vi "Temp Control GUI.vi"(9 "Standalone":bool=TRUE, 10 "Init Data":variant, 11 "Device Name":string="temp control 1") -> ()   [LabVIEW 2024]
uses:
  typedefs/CC enum Operation Mode.ctl
  Subsystems/SS typedef cluster Instrument Command Queue Data.ctl
  Subsystems/SS cluster Data Queue type.ctl
  hk-channel-class/hk-channel-class/HK Item/HK Item.lvclass
  typedefs/CC cluster Alarm Data.ctl
  Temp Control/Temp Control.lvclass
  Current Status/Data Buffer/Data Buffer.lvclass
  typedefs/CC enum Status FG Action.ctl
  Temp Control/Lakeshore 325/Lakeshore 325.lvclass
  Temp Control/Lakeshore 331/Lakeshore 331.lvclass
  Temp Control/Lakeshore 336/Lakeshore 336.lvclass
  Temp Control/Lakeshore 218/Lakeshore 218.lvclass
  typedefs/CC enum Subsystem Status.ctl
  hk-channel-class/hk-channel-class/HK Item/HK Item.lvclass/HK Item.ctl
  hk-channel-class/hk-channel-class/HK Item/HK Channel cluster Telemetry Data.ctl
  hk-channel-class/hk-channel-class/HK Item/HK Channel enum Data Type.ctl
  <vilib>/Utility/error.llb/DialogType.ctl
  hk-channel-class/hk-channel-class/HK Item/Write Source.vi
  6db094d1-7fd6-4988-9962-decbce56bcaa.vi
  40afddd7-fa93-47ab-b467-3e4868690066.vi
panel:
  in  "My Name":string
  in  "Mode":T1
  in  "Tab Control":T2(tab)
  in  "Control enable 2":bool
  in  "Setpoint 2":dbl
  in  "Control enable 1":bool
  in  "Setpoint 1":dbl
  out "Alarm Message":string
  out "Connected":bool
  in  "Status":i32[](listbox)
  out "XY Graph":T3(graph)
  in  "Select Channel":i32=1 min=1 max=4 step=1
  in  "Control Parms":cluster{"P":dbl, "I":dbl, "D":u16}[](array[cluster])
  in  "Reinit":bool
  in  "Heater Range (0: Off)":u16(ring) items=["Off", "Low (0.5W)", "Med (5W)", "High (50W)"]
  in  "Channel Name Prefix":string
  in  "Settings Button":bool
  in  "Power (%)":dbl
  in  "Control Method":bool
  in  "Init Message":string="Connecting to Hardware..."
  in  "Addr":refnum<visa-resource-name>
  in  "Tempcontrol Type":u16(ring) items=["Simulation", "Lakeshore 325", "Lakeshore 336"]
  in  "Close":bool
  out "x-y":u32
  out "Log":string
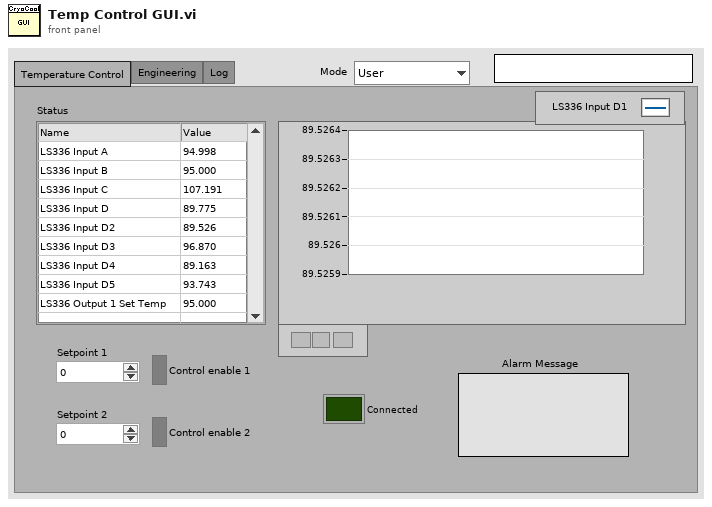
[diagram p1: front panel]
types:
  T1 = typedef "CC enum Operation Mode.ctl" = enum16{"User", "Engineering"}
  T2 = enum32{"Temperature Control", "Engineering", "Log"}
  T3 = cluster{cluster{"Time Stamp":timestamp, "Numeric":dbl}[]}[]
  T4 = typedef "SS typedef cluster Instrument Command Queue Data.ctl" = cluster{"Cmd":string, "Parameters":variant}
  T5 = typedef "CC cluster Alarm Data.ctl" = cluster{"Measured Value":dbl, "Alarm Low":dbl, "Alarm High":dbl, "Message":string, "Source":string}
  T6 = cluster{"state":refnum<user-event>, "cmd q":refnum<queue>, "Cmd":T4, "Data Q":refnum<queue>, "error":errorcluster, "next poll":timestamp, "poll":bool, "Channel List":refnum<class "HK Item.lvclass">[], "Focus Pos":dbl, "Data":dbl[], "Alarm":bool, "Alarms":T5[], "Shutdown":bool, "Device":string, "Temp Control ref":refnum<class "Temp Control.lvclass">, "Buffer":refnum<class "Data Buffer.lvclass">}
  T7 = typedef "CC enum Status FG Action.ctl" = enum16{"Read", "Write", "Init"}
  T8 = typedef "CC enum Subsystem Status.ctl" = enum16{"Unknown", "Ready", "Error"}
  T9 = typedef "SS cluster Data Queue type.ctl" = cluster{"Source":string, "Type":string, "Data":variant}
  T10 = typedef "HK Item.lvclass/HK Channel enum Data Type.ctl" = enum16{"Floating Point", "Integer", "Enum", "String", "Waveform", "File"}
  T11 = typedef "HK Item.lvclass/HK Channel cluster Telemetry Data.ctl" = cluster{"Ch Names":string[], "Ch Values":dbl[], "Timestamp":timestamp, "Data Type":T10}
  T12 = typedef "CC cluster Device Index.ctl" = cluster{"Device Type Name":string, "Curr Device Name":string, "All Instances":string[]}
  T13 = typedef "HK Item.lvclass/HK Channel Units and Setup.ctl" = cluster{"Unit Type":string, "Units":string, "Configuration":string, "Digits":i32, "Data Type":T10, "Exponential?":bool, "Source":string}
  T14 = cluster{cluster{"Time Stamp":timestamp, "Numeric":dbl}[]}
  T15 = typedef "DialogType.ctl" = u16
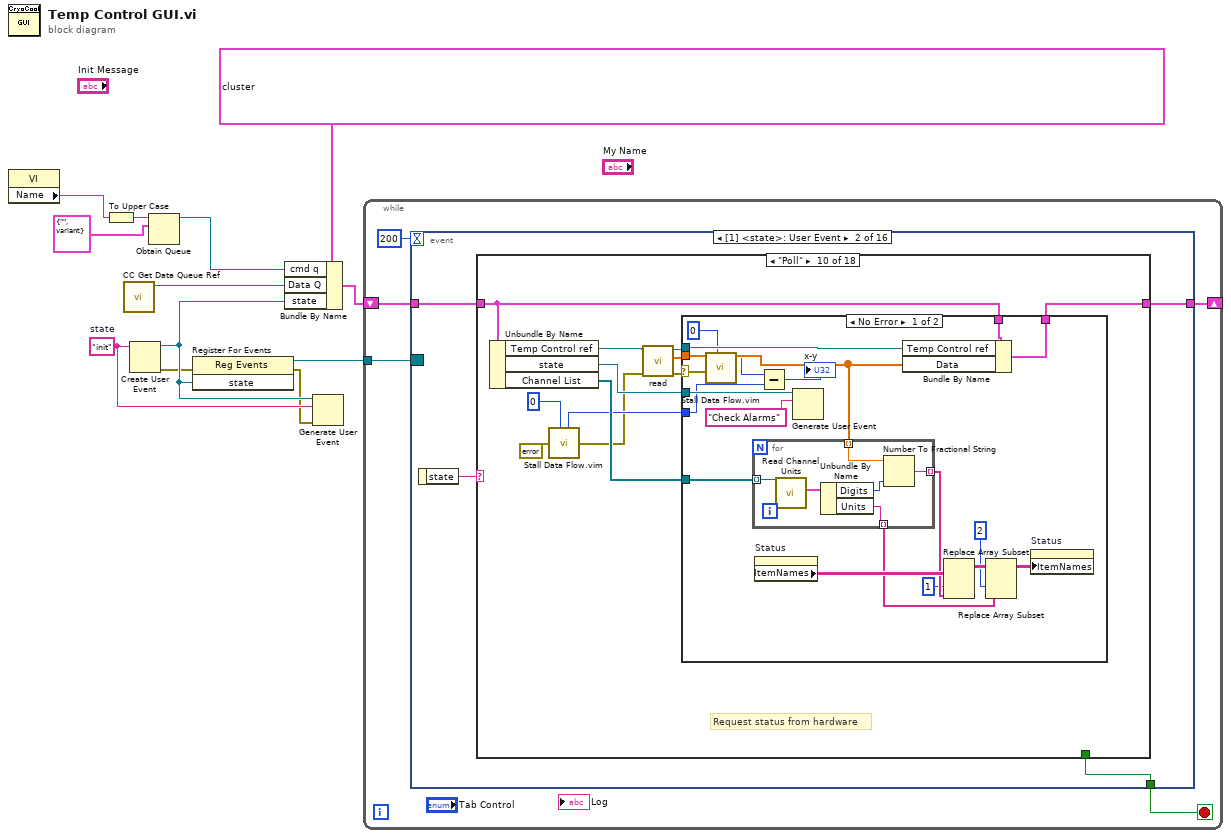
[diagram p0: block diagram]
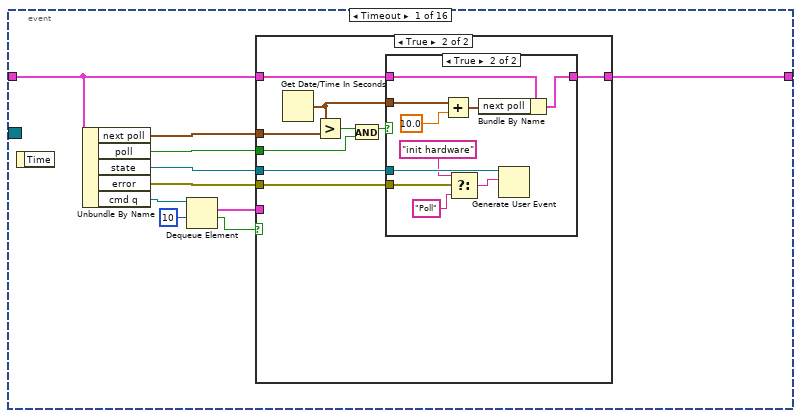
[diagram p2: hidden frame]
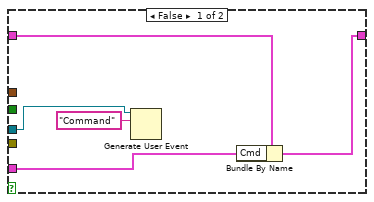
[diagram p3: hidden frame]
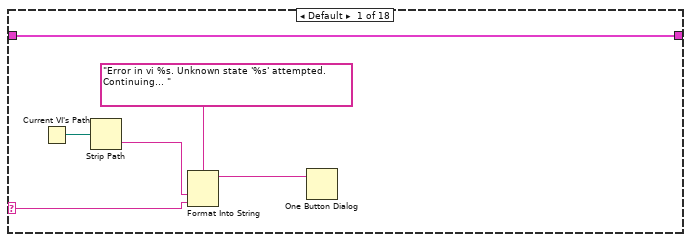
[diagram p5: hidden frame]
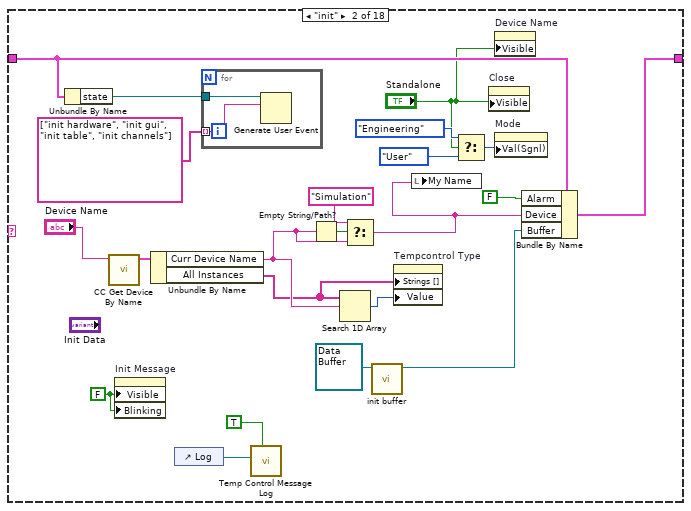
[diagram p6: hidden frame]
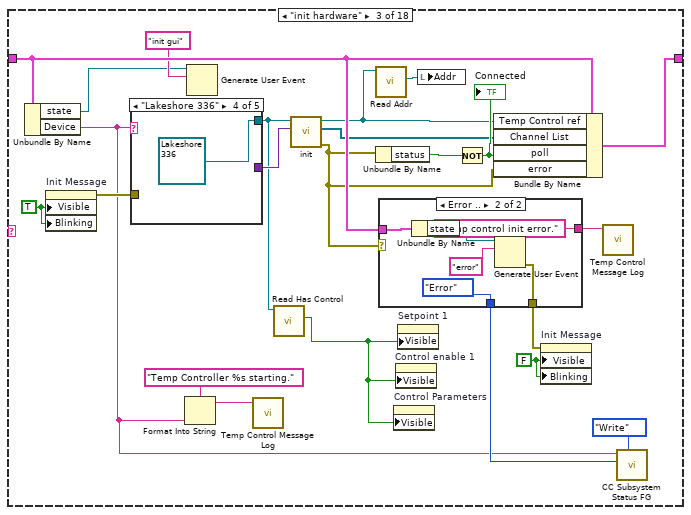
[diagram p7: hidden frame]
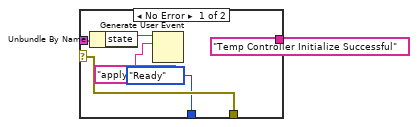
[diagram p8: hidden frame]
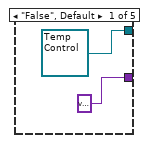
[diagram p9: hidden frame]
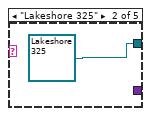
[diagram p10: hidden frame]
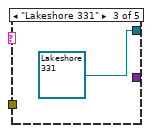
[diagram p11: hidden frame]
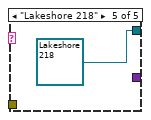
[diagram p12: hidden frame]
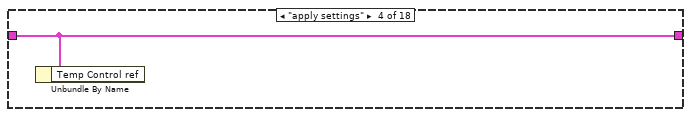
[diagram p13: hidden frame]
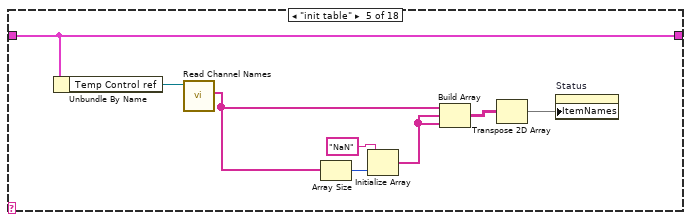
[diagram p14: hidden frame]
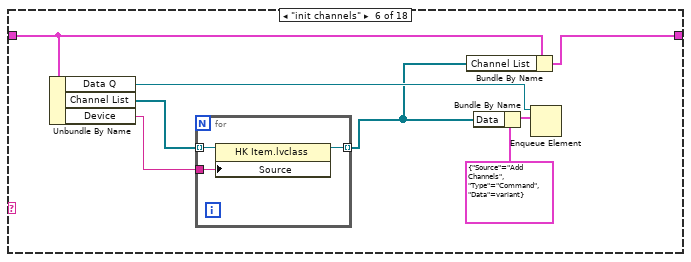
[diagram p15: hidden frame]
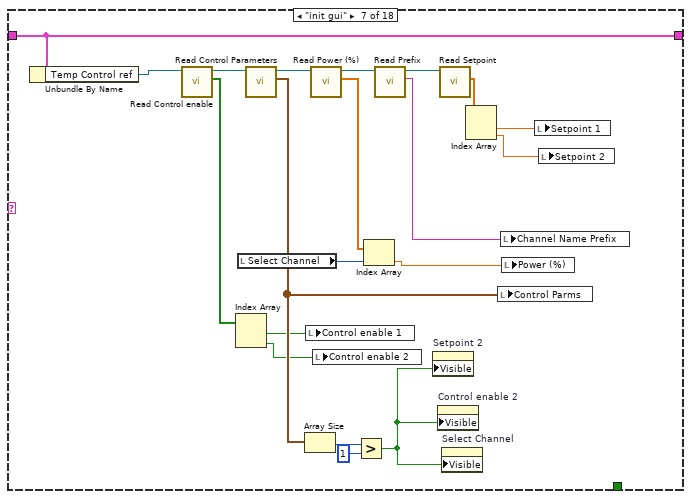
[diagram p16: hidden frame]
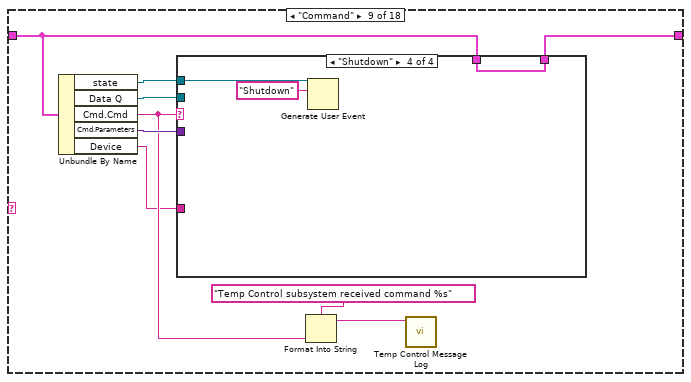
[diagram p18: hidden frame]
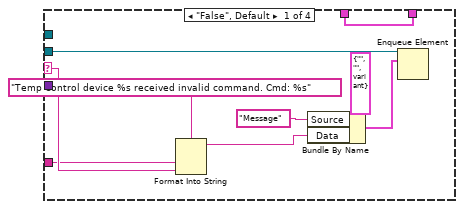
[diagram p19: hidden frame]
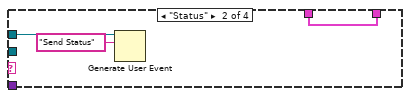
[diagram p20: hidden frame]
diagram:
  w8 = "init"  # state
  n1 = property class="VI"() -> ("Name"=w1:string)  [unwired: 2 in, 2 out]
  n2 = To Upper Case(1:w1) -> (0:w4:string)
  n3 = call "CC Get Data Queue Ref.vi"() -> ("Data Q"=w5:refnum<queue>)  [unwired: 10 in, 1 out]
  n4 = Create User Event(user event datatype=w8) -> (user event=w10:refnum<user-event>, error out=w6:errorcluster)  [unwired: 1 in]
  n5 = Obtain Queue(name (unnamed)=w4, element data type=T4 {"Cmd"="", "Parameters"=variant}) -> (queue out=w2:refnum<queue>)  [unwired: 3 in, 2 out]
  n6 = register-events(error in=w6, w10) -> (reference out=w9:refnum<event-registration>, error out=w7:errorcluster)  [unwired: 1 in]
  n7 = Bundle By Name(cluster=T6 {"state"=refnum, "cmd q"=refnum, "Cmd"={"Cmd"="", "Parameters"=variant}, "Data Q"=refnum, "error"={"status"=FALSE, "code"=0, "source"=""}, "next poll"=timestamp(0 s since 1904-01-01), "poll"=FALSE, "Channel List"=[], "Focus Pos"=0.0, "Data"=[], "Alarm"=FALSE, "Alarms"=[], "Shutdown"=FALSE, "Device"="", "Temp Control ref"=refnum, "Buffer"=refnum}, "cmd q"=w2, "Data Q"=w5, "state"=w10) -> (w11:T6)
  n8 = Generate User Event(user event=w10, event data cluster=w8, error in=w7) -> ()  [unwired: 1 in, 2 out]
  n9 = while {
    tunnel: w9 -> [w17]
    shift-right: [w15] -> _
    shift-left: w11 -> [w16]
    stop <- w14 stop-if-true
    n10 = event shown="[1] <state>: User Event" {
      selector: w17 -> [_ _ _ _ _ _ _ _ _ _ _ _ _ _ _ _]
      dyn-events: _ -> [_ _ _ _ _ _ _ _ _ _ _ _ _ _ _ _]
      timeout: 200 -> [_ _ _ _ _ _ _ _ _ _ _ _ _ _ _ _]
      tunnel: w16 -> [w22 w55 w314 w318 w323 w333 w345 w358 w374 w381 w382 w406 w411 w418 w424 w431]
      tunnel: [w21 w54 w314 w319 w324 w334 w346 w359 w375 w381 w383 w407 w412 w418 w424 w431] -> w15
      tunnel: [_ w53 _ _ _ _ _ _ _ _ _ _ _ _ _ _] -> w14
      event Timeout {
        n11 = event-data() -> ()  [unwired: 1 in, 1 out]
        n12 = Unbundle By Name(w22) -> ("next poll"=w20:timestamp, "poll"=w19:bool, "state"=w23:refnum<user-event>, "error"=w18:errorcluster, "cmd q"=w27:refnum<queue>)
        n13 = Dequeue Element(queue=w27, timeout in ms (-1)=10) -> (element=w24:T4, timed out?=w25:bool)  [unwired: 1 in, 2 out]
        n14 = case shown="True" w25 {
          tunnel: w24 -> [w29 _]
          tunnel: w23 -> [w32 w38]
          tunnel: w22 -> [w30 w39]
          tunnel: [w28 w36] -> w21
          tunnel: w20 -> [_ w41]
          tunnel: w19 -> [_ w34]
          tunnel: w18 -> [_ w33]
          frame False {
            n15 = Generate User Event(user event=w32, event data cluster="Command" ("event data")) -> ()  [unwired: 2 in, 2 out]
            n16 = Bundle By Name(cluster=w30, "Cmd"=w29) -> (w28:T6)
          }
          frame True {
            n17 = Get Date/Time In Seconds() -> (seconds since 1Jan1904=w37:timestamp)
            n18 = Greater?(x=w37, y=w41) -> (0:w40:bool)
            n19 = And(x=w40, y=w34) -> (x .and. y?=w35:bool)
            n20 = case shown="True" w35 {
              tunnel: w39 -> [w42 w52]
              tunnel: w38 -> [_ w51]
              tunnel: w37 -> [_ w50]
              tunnel: [w42 w47] -> w36
              tunnel: w33 -> [_ w45]
              frame False {
              }
              frame True {
                n21 = Add(x=w50, y=10.0) -> (x+y=w48:timestamp)
                n22 = Select(t="init hardware", s=w45, f="Poll" ("event data")) -> (s? t:f=w43:string)
                n23 = Bundle By Name(cluster=w52, "next poll"=w48) -> (w47:T6)
                n24 = Generate User Event(user event=w51, event data cluster=w43) -> ()  [unwired: 2 in, 2 out]
              }
            }
          }
        }
      }
      event User Event {
        n25 = event-data() -> ("state"=w56:string)  [unwired: 1 in]
        n26 = case shown="\"Poll\"" w56 {
          selector: w56 -> [w61 _ _ _ _ _ _ _ _ _ _ _ _ _ _ _ _ _]
          tunnel: w55 -> [w57 w82 w106 w128 w136 w138 w167 w168 w173 w206 w239 w245 w253 w258 w275 w282 w286 w310]
          tunnel: [w57 w83 w109 w128 w136 w139 w167 w168 w174 w207 w239 w245 w253 w258 w275 w283 w287 w310] -> w54
          tunnel: [_ _ _ _ _ _ _ _ _ _ _ _ _ _ _ _ _ TRUE] -> w53
          frame Default {
            n27 = Current VI's Path() -> (path=w60:path)
            n28 = Strip Path(path=w60) -> (name=w59:string)  [unwired: 1 out]
            n29 = Format Into String(format string="Error in vi %s. Unknown state '%s' attempted. Continuing... ", w59, w61) -> (resulting string=w58:string)  [unwired: 2 in, 1 out]
            n30 = One Button Dialog(message=w58) -> ()  [unwired: 1 in, 1 out]
          }
          frame "init" {
            w69 = FALSE ("Visible")
            n31 = Unbundle By Name(w82) -> ("state"=w81:refnum<user-event>)
            n32 = call "CC Get Device By Name.vi"("Device Type"="Device Name") -> ("Device"=w77:T12)  [unwired: 8 in, 2 out]
            n33 = property on="Init Message" class="Str"("Visible"=w69, "Blinking"=w69) -> ()  [unwired: 2 in, 2 out]
            n34 = Unbundle By Name(w77) -> ("Curr Device Name"=w76:string, "All Instances"=w75:string[])
            n35 = control-ref of="Log"() -> (w71:refnum<vi>)
            n36 = for {
              tunnel: w81 -> [w86]
              tunnel: string[] ["init hardware", "init gui", "init table", "init channels"] -> [w85] mode=indexing
              n37 = Generate User Event(user event=w86, event data cluster=w85) -> ()  [unwired: 2 in, 2 out]
            }
            n38 = call "Temp Control Message Log.vi"("init?"=TRUE, "Log Ref"=w71) -> ()  [unwired: 8 in, 2 out]
            n39 = Empty String/Path?(string/path=w76) -> (empty?=w84:bool)
            n40 = Search 1D Array(1D array=w75, element=w76) -> (index of element=w79:i32)  [unwired: 1 in]
            n41 = Select(t="Simulation", s=w84, f=w76) -> (s? t:f=w67:string)
            n42 = call-dynamic "init buffer.vi"("Data Buffer in"=refnum<class "Data Buffer.lvclass"> refnum) -> ("Data Buffer out"=w65:refnum<class "Data Buffer.lvclass">)  [unwired: 9 in, 1 out]
            n43 = property on="Tempcontrol Type" class="Ring (strict)"("Strings []"=w75, "Value"=w79) -> ()  [unwired: 2 in, 2 out]
            n44 = local write "My Name"(w67) -> ()
            n45 = Select(t=CC_enum_Operation_Mode."Engineering" ("Mode"), s="Standalone", f=CC_enum_Operation_Mode."User" ("Mode")) -> (s? t:f=w72:T1)
            n46 = property on="Close" class="Bool"("Visible"="Standalone") -> ()  [unwired: 2 in, 2 out]
            n47 = property on="Device Name" class="Str"("Visible"="Standalone") -> ()  [unwired: 2 in, 2 out]
            n48 = property on="Mode" class="Enum (strict)"("Val(Sgnl)"=w72) -> ()  [unwired: 2 in, 2 out]
            n49 = Bundle By Name(cluster=w82, "Alarm"=FALSE, "Device"=w67, "Buffer"=w65) -> (w83:T6)
          }
          frame "init hardware" {
            w101 = FALSE ("Visible")
            w103 = TRUE ("Visible")
            n50 = Unbundle By Name(w106) -> ("state"=w87:refnum<user-event>, "Device"=w94:string)
            n51 = property on="Init Message" class="Str"("Visible"=w103, "Blinking"=w103) -> (error out=w102:errorcluster)  [unwired: 2 in, 1 out]
            n52 = case shown="\"Lakeshore 336\"" w94 {
              tunnel: [refnum<class "Temp Control.lvclass"> refnum ("Temp Control.lvclass") refnum<class "Lakeshore 325.lvclass"> refnum ("Lakeshore 325.lvclass") refnum<class "Lakeshore 331.lvclass"> refnum ("Lakeshore 331.lvclass") refnum<class "Lakeshore 336.lvclass"> refnum ("Lakeshore 336.lvclass") refnum<class "Lakeshore 218.lvclass"> refnum ("Lakeshore 218.lvclass")] -> w91
              tunnel: [variant _ _ _ _] -> w95
              tunnel: w102 -> [_ _ _ _ _]
              frame "False", Default {
              }
              frame "Lakeshore 325" {
              }
              frame "Lakeshore 331" {
              }
              frame "Lakeshore 336" {
              }
              frame "Lakeshore 218" {
              }
            }
            n53 = Format Into String(format string="Temp Controller %s starting.", w94) -> (resulting string=w104:string)  [unwired: 2 in, 1 out]
            n54 = Generate User Event(user event=w87, event data cluster="init gui" ("event data")) -> ()  [unwired: 2 in, 2 out]
            n55 = call "Temp Control Message Log.vi"("String in"=w104) -> ()  [unwired: 9 in, 2 out]
            n56 = call-dynamic "Read Has Control.vi"("Temp Control in"=w91) -> ("Has Control"=w90:bool)  [unwired: 8 in, 2 out]
            n57 = call-dynamic "init.vi"("Init Data"=w95, "Temp Control in"=w91) -> ("error out"=w96:errorcluster, "Channel List"=w97:refnum<class "HK Item.lvclass">[], "Temp Control out"=w92:refnum<class "Temp Control.lvclass">)  [unwired: 7 in]
            n58 = call-dynamic "Read Addr.vi"("Temp Control in"=w92) -> ("Addr"=w93:refnum<visa-resource-name>)  [unwired: 8 in, 2 out]
            n59 = Unbundle By Name(w96) -> ("status"=w108:bool)
            n60 = case shown="Error .." w96 {
              selector: w96 -> [w115 _]
              tunnel: w106 -> [w112 w121]
              tunnel: [w115 w118] -> w100
              tunnel: [CC_enum_Subsystem_Status."Ready" ("Status") CC_enum_Subsystem_Status."Error" ("Status")] -> w98
              tunnel: ["Temp Controller Initialize Successful" ("String in") "Temp control init error." ("String in")] -> w88
              frame No Error {
                n61 = Unbundle By Name(w112) -> ("state"=w111:refnum<user-event>)
                n62 = Generate User Event(user event=w111, event data cluster="apply settings" ("event data")) -> ()  [unwired: 2 in, 2 out]
              }
              frame Error {
                n63 = Unbundle By Name(w121) -> ("state"=w120:refnum<user-event>)
                n64 = Generate User Event(user event=w120, event data cluster="error" ("event data")) -> (error out=w118:errorcluster)  [unwired: 2 in, 1 out]
              }
            }
            n65 = property on="Control Parameters" class="Clust (strict)"("Visible"=w90) -> ()  [unwired: 2 in, 2 out]
            n66 = property on="Control enable 1" class="Bool (strict)"("Visible"=w90) -> ()  [unwired: 2 in, 2 out]
            n67 = property on="Setpoint 1" class="DigNum (strict)"("Visible"=w90) -> ()  [unwired: 2 in, 2 out]
            n68 = local write "Addr"(w93) -> ()
            n69 = Not(x=w108) -> (.not. x?=w105:bool)
            "Connected" <- w105
            n70 = Bundle By Name(cluster=w106, "Temp Control ref"=w92, "Channel List"=w97, "poll"=w105, "error"=w96) -> (w109:T6)
            n71 = property on="Init Message" class="Str"(error in=w100, "Visible"=w101, "Blinking"=w101) -> ()  [unwired: 1 in, 2 out]
            n72 = call "Temp Control Message Log.vi"("String in"=w88) -> ()  [unwired: 9 in, 2 out]
            n73 = call "CC Subsystem Status FG.vi"("Action"=CC_enum_Status_FG_Action."Write", "Status"=w98, "Subsystem Name"=w94) -> ()  [unwired: 7 in, 2 out]
          }
          frame "apply settings" {
            n74 = Unbundle By Name(w128) -> ()  [unwired: 1 out]
          }
          frame "init table" {
            n75 = Unbundle By Name(w136) -> ("Temp Control ref"=w130:refnum<class "Temp Control.lvclass">)
            n76 = call-dynamic "Read Channel Names.vi"("Temp Control in"=w130) -> ("Channel Names"=w129:string[])  [unwired: 8 in, 2 out]
            n77 = Array Size(array=w129) -> (size(s)=w135:i32)
            n78 = Initialize Array("NaN", w135) -> (w131:string[])
            n79 = Build Array(w129, w131, w131) -> (w133:string[][])
            n80 = Transpose 2D Array(2D array=w133) -> (transposed array=w132:string[][])
            n81 = property on="Status" class="MCListbox (strict)"("ItemNames"=w132) -> ()  [unwired: 2 in, 2 out]
          }
          frame "init channels" {
            n82 = Unbundle By Name(w138) -> ("Data Q"=w142:refnum<queue>, "Channel List"=w141:refnum<class "HK Item.lvclass">[], "Device"=w137:string)
            n83 = for {
              tunnel: w141 -> [w147] mode=indexing
              tunnel: [w146] -> w140 mode=indexing
              tunnel: w137 -> [w145]
              n84 = property class="HK Item.lvclass"(reference=w147, "Source"=w145) -> (reference out=w146:refnum<class "HK Item.lvclass">)  [unwired: 1 in, 1 out]
            }
            n85 = Bundle By Name(cluster=w138, "Channel List"=w140) -> (w139:T6)
            n86 = Bundle By Name(cluster=T9 {"Source"="Add Channels", "Type"="Command", "Data"=variant} ("element"), "Data"=w140) -> (w144:T9)
            n87 = Enqueue Element(queue=w142, element=w144) -> ()  [unwired: 2 in, 3 out]
          }
          frame "init gui" {
            n88 = Unbundle By Name(w167) -> ("Temp Control ref"=w166:refnum<class "Temp Control.lvclass">)
            n89 = call-dynamic "Read Control enable.vi"("Temp Control in"=w166) -> ("Control Enable"=w160:bool[], "Temp Control out"=w165:refnum<class "Temp Control.lvclass">)  [unwired: 8 in, 1 out]
            n90 = Index Array(array=w160) -> (element #1=w154:bool, element #2=w148:bool)  [unwired: 2 in]
            n91 = local read "Select Channel"() -> (w150:i32)
            n92 = call-dynamic "Read Control Parameters.vi"("Temp Control in"=w165) -> ("Control Parameters"=w158:cluster{"P":dbl, "I":dbl, "D":u16}[], "Temp Control out"=w164:refnum<class "Temp Control.lvclass">)  [unwired: 8 in, 1 out]
            n93 = Array Size(array=w158) -> (size(s)=w157:i32)
            n94 = local write "Control enable 1"(w154) -> ()
            n95 = call-dynamic "Read Power (%).vi"("Temp Control in"=w164) -> ("Power (%)"=w153:dbl[], "Temp Control out"=w163:refnum<class "Temp Control.lvclass">)  [unwired: 8 in, 1 out]
            n96 = local write "Control enable 2"(w148) -> ()
            n97 = Greater?(x=w157, y=1) -> (0:w155:bool)
            n98 = Index Array(array=w153, index=w150) -> (element=w152:dbl)
            n99 = call-dynamic "Read Prefix.vi"("Temp Control in"=w163) -> ("Prefix"=w161:string, "Temp Control out"=w162:refnum<class "Temp Control.lvclass">)  [unwired: 8 in, 1 out]
            n100 = property on="Setpoint 2" class="DigNum (strict)"("Visible"=w155) -> ()  [unwired: 2 in, 2 out]
            n101 = property on="Control enable 2" class="Bool (strict)"("Visible"=w155) -> ()  [unwired: 2 in, 2 out]
            n102 = call-dynamic "Read Setpoint.vi"("Temp Control in"=w162) -> ("Setpoint"=w159:dbl[])  [unwired: 8 in, 2 out]
            n103 = property on="Select Channel" class="DigNum (strict)"("Visible"=w155) -> ()  [unwired: 2 in, 2 out]
            n104 = Index Array(array=w159) -> (element #1=w151:dbl, element #2=w149:dbl)  [unwired: 2 in]
            n105 = local write "Control Parms"(w158) -> ()
            n106 = local write "Channel Name Prefix"(w161) -> ()
            n107 = local write "Power (%)"(w152) -> ()
            n108 = local write "Setpoint 1"(w151) -> ()
            n109 = local write "Setpoint 2"(w149) -> ()
          }
          frame "send command" {
          }
          frame "Command" {
            n110 = Unbundle By Name(w173) -> ("state"=w175:refnum<user-event>, "Data Q"=w177:refnum<queue>, "Cmd.Cmd"=w171:string, "Cmd.Parameters"=w176:variant, "Device"=w169:string)
            n111 = case shown="\"Shutdown\"" w171 {
              selector: w171 -> [w179 _ _ _]
              tunnel: w177 -> [w186 _ _ _]
              tunnel: w176 -> [_ _ _ _]
              tunnel: w175 -> [_ w189 w191 w195]
              tunnel: w173 -> [w180 w187 w190 w193]
              tunnel: [w180 w187 w190 w193] -> w174
              tunnel: w169 -> [w178 _ _ _]
              frame "False", Default {
                n112 = Format Into String(format string="Temp Control device %s received invalid command. Cmd: %s", w178, w179) -> (resulting string=w182:string)  [unwired: 2 in, 1 out]
                n113 = Bundle By Name(cluster=T9 {"Source"="", "Type"="", "Data"=variant} ("element"), "Source"="Message" ("Data Type"), "Data"=w182) -> (w181:T9)
                n114 = Enqueue Element(queue=w186, element=w181) -> ()  [unwired: 2 in, 3 out]
              }
              frame "Status" {
                n115 = Generate User Event(user event=w189, event data cluster="Send Status" ("event data")) -> ()  [unwired: 2 in, 2 out]
              }
              frame "Config" {
                n116 = Generate User Event(user event=w191, event data cluster="Send Config" ("event data")) -> ()  [unwired: 2 in, 2 out]
              }
              frame "Shutdown" {
                n117 = Generate User Event(user event=w195, event data cluster="Shutdown" ("event data")) -> ()  [unwired: 2 in, 2 out]
              }
            }
            n118 = Format Into String(format string="Temp Control subsystem received command %s", w171) -> (resulting string=w170:string)  [unwired: 2 in, 1 out]
            n119 = call "Temp Control Message Log.vi"("String in"=w170) -> ()  [unwired: 9 in, 2 out]
          }
          frame "Poll" {
            # "Request status from hardware"
            n120 = Unbundle By Name(w206) -> ("Temp Control ref"=w200:refnum<class "Temp Control.lvclass">, "state"=w205:refnum<user-event>, "Channel List"=w204:refnum<class "HK Item.lvclass">[])
            n121 = call "Stall Data Flow.vim"("value in"=errorcluster {"status"=FALSE, "code"=0, "source"=""} ("error in (no error)"), "milliseconds to wait"=u32 0) -> ("millisecond timer value"=w201:u32, "value out"=w199:errorcluster)
            n122 = call-dynamic "read.vi"("error in (no error)"=w199, "Temp Control in"=w200) -> ("error out"=w196:errorcluster, "Data"=w197:dbl[], "Temp Control out"=w198:refnum<class "Temp Control.lvclass">)  [unwired: 7 in]
            n123 = case shown="No Error" w196 {
              selector: w196 -> [w216 w234]
              tunnel: [w226 w233] -> w207
              tunnel: w206 -> [w225 w235]
              tunnel: w205 -> [w224 w237]
              tunnel: w198 -> [w222 _]
              tunnel: w204 -> [w221 _]
              tunnel: w197 -> [w220 _]
              tunnel: w201 -> [w213 _]
              frame No Error {
                n124 = call "Stall Data Flow.vim"("value in"=w216, "milliseconds to wait"=u32 0) -> ("millisecond timer value"=w214:u32)  [unwired: 1 out]
                n125 = for {
                  tunnel: w221 -> [w232] mode=indexing
                  tunnel: w220 -> [w229] mode=indexing
                  tunnel: [w228] -> w218 mode=indexing
                  tunnel: [w227] -> w209 mode=indexing
                  n126 = call "Read Channel Units.vi"("HK Item in"=w232) -> ("Channel Setup"=w231:T13)  [unwired: 8 in, 2 out]
                  n127 = Unbundle By Name(w231) -> ("Digits"=w230:i32, "Units"=w227:string)
                  n128 = Number To Fractional String(number=w229, precision (6)=w230) -> (F-format string=w228:string)  [unwired: 2 in]
                }
                n129 = property on="Status" class="MCListbox (strict)"() -> ("ItemNames"=w219:string[][])  [unwired: 2 in, 2 out]
                n130 = Subtract(x=w214, y=w213) -> (x-y=→"x-y":u32)
                n131 = Generate User Event(user event=w224, event data cluster="Check Alarms" ("event data")) -> ()  [unwired: 2 in, 2 out]
                n132 = Bundle By Name(cluster=w225, "Temp Control ref"=w222, "Data"=w220) -> (w226:T6)
                n133 = Replace Array Subset(array=w219, new element=w218, index (col)=1 ("disabled index (col)")) -> (w211:string[][])  [unwired: 1 in]
                n134 = Replace Array Subset(array=w211, new element=w209, index (col)=2 ("disabled index (col)")) -> (w208:string[][])  [unwired: 1 in]
                n135 = property on="Status" class="MCListbox (strict)"("ItemNames"=w208) -> ()  [unwired: 2 in, 2 out]
              }
              frame Error {
                n136 = Generate User Event(user event=w237, event data cluster="error" ("event data")) -> ()  [unwired: 2 in, 2 out]
                n137 = Bundle By Name(cluster=w235, "error"=w234) -> (w233:T6)
              }
            }
          }
          frame "Check Alarms" {
            n138 = Unbundle By Name(w239) -> ("state"=w238:refnum<user-event>)
            n139 = Generate User Event(user event=w238, event data cluster="Send Status" ("event data")) -> ()  [unwired: 2 in, 2 out]
          }
          frame "Alarm Set" {
            n140 = Unbundle By Name(w245) -> ("Data Q"=w250:refnum<queue>, "Device"=w242:string, "Alarms"=w247:T5[])
            n141 = Index Array(array=w247) -> (element=w246:T5)  [unwired: 1 in]
            n142 = Bundle By Name(cluster=w246, "Source"=w242) -> (w243:T5)
            n143 = Unbundle By Name(w243) -> ("Message"=w244:string)
            "Alarm Message" <- w244
            n144 = Bundle By Name(cluster=T9 {"Source"="", "Type"="", "Data"=variant} ("element"), "Source"=w242, "Type"="Alarm Set", "Data"=w243) -> (w241:T9)
            n145 = Enqueue Element(queue=w250, element=w241) -> ()  [unwired: 2 in, 3 out]
            n146 = call "Temp Control Message Log.vi"("String in"=w244) -> ()  [unwired: 9 in, 2 out]
          }
          frame "Alarm Clear" {
            n147 = Unbundle By Name(w253) -> ("Data Q"=w257:refnum<queue>, "Device"=w254:string)
            n148 = Bundle By Name(cluster=T9 {"Source"="", "Type"="", "Data"=variant} ("element"), "Source"=w254, "Type"="Alarm Clear") -> (w251:T9)
            n149 = call "Temp Control Message Log.vi"("String in"="Alarm condition cleared.") -> ()  [unwired: 9 in, 2 out]
            n150 = Enqueue Element(queue=w257, element=w251) -> ()  [unwired: 2 in, 3 out]
          }
          frame "Alarm Shutdown" {
          }
          frame "Send Status" {
            n151 = Unbundle By Name(w275) -> ("Data Q"=w274:refnum<queue>, "Device"=w264:string, "Temp Control ref"=w263:refnum<class "Temp Control.lvclass">, "Data"=w260:dbl[], "Buffer"=w261:refnum<class "Data Buffer.lvclass">)
            n152 = call-dynamic "Read Channel Names.vi"("Temp Control in"=w263) -> ("Channel Names"=w262:string[])  [unwired: 8 in, 2 out]
            n153 = Get Date/Time In Seconds() -> (seconds since 1Jan1904=w267:timestamp)
            n154 = call-dynamic "write buffer.vi"("Data"=w260, "Data Buffer in"=w261) -> ("XY Graph"=w259:T3)  [unwired: 7 in, 2 out]
            n155 = Bundle(cluster=T11 {"Ch Names"=[], "Ch Values"=[], "Timestamp"=timestamp(0 s since 1904-01-01), "Data Type"=enum."Floating Point"}, "Ch Names"=w262, "Ch Values"=w260, "Timestamp"=w267, "Data Type"=HK_Channel_enum_Data_Type."Floating Point") -> (w269:T11)
            n156 = for {
              tunnel: "Status" -> [w277] mode=indexing
              tunnel: w259 -> [w278]
              tunnel: [w276] -> w265 mode=indexing
              n157 = Index Array(array=w278, index=w277) -> (element=w276:T14)
            }
            "XY Graph" <- w265
            n158 = Bundle By Name(cluster=T9 {"Source"="", "Type"="", "Data"=variant} ("element"), "Source"=w264, "Type"="Floating Point" ("Data Type"), "Data"=w269) -> (w271:T9)
            n159 = Enqueue Element(queue=w274, element=w271) -> ()  [unwired: 2 in, 3 out]
          }
          frame "Reinit" {
            n160 = Unbundle By Name(w282) -> ("Temp Control ref"=w281:refnum<class "Temp Control.lvclass">, "state"=w285:refnum<user-event>)
            n161 = call-dynamic "close.vi"("Temp Control in"=w281) -> ("error out"=w279:errorcluster, "Temp Control out"=w280:refnum<class "Temp Control.lvclass">)  [unwired: 9 in]
            n162 = Generate User Event(user event=w285, event data cluster="init hardware" ("event data")) -> ()  [unwired: 2 in, 2 out]
            n163 = call <vilib>:"Clear Errors.vi"("error in (no error)"=w279) -> ()  [unwired: 5 in, 2 out]
            n164 = Bundle By Name(cluster=w282, "Temp Control ref"=w280) -> (w283:T6)
          }
          frame "error" {
            w299 = T15 0 items=["no dialog", "OK message", "continue or stop message", "OK message + warnings", "continue/stop + warnings"] ("type of dialog (OK msg:1)")
            n165 = Unbundle By Name(w286) -> ("Device"=w291:string, "error"=w302:errorcluster, "error.code"=w305:i32, "error.source"=w303:string, "Data Q"=w293:refnum<queue>)
            n166 = call <vilib>:"Simple Error Handler.vi"("type of dialog (OK msg:1)"=w299, "error in (no error)"=w302) -> ("message"=w301:string)  [unwired: 3 in, 4 out]
            n167 = Bundle By Name(cluster=T5 {"Measured Value"=0.0, "Alarm Low"=0.0, "Alarm High"=0.0, "Message"="", "Source"=""} ("element"), "Source"=w291, "Message"="Temp Controller Initialization Error. Check Communications port.") -> (w295:T5)
            n168 = Format Into String(format string="Error from Temperature Controller \"%s\". Error # %d, Error Source: %s, Error message \"%s\"", w291, w305, w303, w301) -> (resulting string=w300:string)  [unwired: 2 in, 1 out]
            n169 = Bundle By Name(cluster=T9 {"Source"="", "Type"="", "Data"=variant} ("element"), "Source"=w291, "Type"="Alarm Set", "Data"=w295) -> (w292:T9)
            n170 = call "Temp Control Message Log.vi"("String in"=w300) -> ()  [unwired: 9 in, 2 out]
            n171 = Get Date/Time In Seconds() -> (seconds since 1Jan1904=w290:timestamp)
            n172 = Add(x=w290, y=120.0) -> (x+y=w288:timestamp)
            n173 = Enqueue Element(queue=w293, element=w292) -> ()  [unwired: 2 in, 3 out]
            n174 = Bundle By Name(cluster=w286, "next poll"=w288) -> (w287:T6)
          }
          frame "Shutdown" {
            n175 = Unbundle By Name(w310) -> ("Data Q"=w309:refnum<queue>, "Temp Control ref"=w307:refnum<class "Temp Control.lvclass">)
            n176 = Release Queue(queue=w309) -> ()  [unwired: 2 in, 3 out]
            n177 = call-dynamic "close.vi"("Temp Control in"=w307) -> ("error out"=w306:errorcluster)  [unwired: 9 in, 1 out]
            n178 = call <vilib>:"Clear Errors.vi"("error in (no error)"=w306) -> ()  [unwired: 5 in, 2 out]
            n179 = call "Temp Control Message Log.vi"("String in"="Temp Control shutting down.") -> ()  [unwired: 9 in, 2 out]
          }
        }
      }
      event "Select Channel": Value Change {
        n180 = event-data() -> ()  [unwired: 1 in, 1 out]
        n181 = Unbundle By Name(w314) -> ("state"=w313:refnum<user-event>)
        n182 = Generate User Event(user event=w313, event data cluster="init gui" ("event data")) -> ()  [unwired: 2 in, 2 out]
      }
      event "Channel Name Prefix": Value Change {
        n183 = event-data() -> ()  [unwired: 1 in, 6 out]
        n184 = Unbundle By Name(w318) -> ("Temp Control ref"=w321:refnum<class "Temp Control.lvclass">)
        n185 = call-dynamic "Write Prefix.vi"("Prefix"="Channel Name Prefix", "Temp Control in"=w321) -> ("Temp Control out"=w317:refnum<class "Temp Control.lvclass">)  [unwired: 8 in, 1 out]
        n186 = call-dynamic "Read Channel List.vi"("Temp Control in"=w317) -> ("Channel List"=w315:refnum<class "HK Item.lvclass">[], "Temp Control out"=w316:refnum<class "Temp Control.lvclass">)  [unwired: 8 in, 1 out]
        n187 = Bundle By Name(cluster=w318, "Temp Control ref"=w316, "Channel List"=w315) -> (w319:T6)
      }
      event "Control Parms": Value Change {
        n188 = event-data() -> ()  [unwired: 1 in, 6 out]
        n189 = Unbundle By Name(w323) -> ("Temp Control ref"=w326:refnum<class "Temp Control.lvclass">)
        n190 = call-dynamic "Set PID.vi"("Control Parameters"="Control Parms", "Temp Control in"=w326) -> ("Temp Control out"=w325:refnum<class "Temp Control.lvclass">)  [unwired: 8 in, 1 out]
        n191 = Bundle By Name(cluster=w323, "Temp Control ref"=w325) -> (w324:T6)
      }
      event "Control Method", "Power (%)", "Heater Range (0: Off)": Value Change {
        n192 = event-data() -> ()  [unwired: 1 in, 6 out]
        n193 = Unbundle By Name(w333) -> ("Temp Control ref"=w337:refnum<class "Temp Control.lvclass">)
        n194 = call-dynamic "Set Manual Mode.vi"("Heater Range (0: Off)"="Heater Range (0: Off)", "Channel (1)"="Select Channel", "Power"="Power (%)", "Manual Mode"="Control Method", "Temp Control in"=w337) -> ("Temp Control out"=w335:refnum<class "Temp Control.lvclass">)  [unwired: 5 in, 1 out]
        n195 = Bundle By Name(cluster=w333, "Temp Control ref"=w335) -> (w334:T6)
        n196 = case shown="False" "Control Method" {
          tunnel: ["manual" "auto"] -> w327
          frame False {
          }
          frame True {
            n197 = local write "Control enable 1"(FALSE ("Control enable")) -> ()
          }
        }
        n198 = Format Into String(format string="Temperature control channel %d set to %s", "Select Channel", w327) -> (resulting string=w329:string)  [unwired: 2 in, 1 out]
        n199 = call "Temp Control Message Log.vi"("String in"=w329) -> ()  [unwired: 9 in, 2 out]
      }
      event "Settings Button": Value Change {
        n200 = event-data() -> ()  [unwired: 1 in, 6 out]
        n201 = Unbundle By Name(w345) -> ("Temp Control ref"=w347:refnum<class "Temp Control.lvclass">)
        n202 = call-dynamic "Set Parameters GUI.vi"("Temp Control in"=w347) -> ("Temp Control out"=w344:refnum<class "Temp Control.lvclass">)  [unwired: 9 in, 1 out]
        n203 = call-dynamic "Read Control Parameters.vi"("Temp Control in"=w344) -> ("Control Parameters"=w342:cluster{"P":dbl, "I":dbl, "D":u16}[], "Temp Control out"=w343:refnum<class "Temp Control.lvclass">)  [unwired: 8 in, 1 out]
        n204 = Array Size(array=w342) -> (size(s)=w341:i32)
        n205 = Bundle By Name(cluster=w345, "Temp Control ref"=w343) -> (w346:T6)
        n206 = property on="Control Parms" class="Arr (strict)"("Number of Rows"=w341, "Value"=w342) -> ()  [unwired: 2 in, 2 out]
      }
      event "Control enable 1", "Control enable 2": Value Change {
        n207 = event-data() -> ("CtlRef"=w356:refnum<vi>)  [unwired: 1 in, 5 out]
        n208 = property class="Bool (strict)"(reference=w356) -> ("Label.Text"=w355:string)  [unwired: 1 in, 2 out]
        n209 = local write "Control Method"(FALSE ("Manual Control")) -> ()
        n210 = case shown="\"False\", Default" w355 {
          tunnel: ["Control enable 1" "Control enable 2"] -> w351
          tunnel: [1 ("Select Channel") 2 ("Select Channel")] -> w352
          frame "False", Default {
          }
          frame "Control enable 2" {
          }
        }
        n211 = Unbundle By Name(w358) -> ("Temp Control ref"=w361:refnum<class "Temp Control.lvclass">)
        n212 = Select(t="enabled", s=w351, f="disabled") -> (s? t:f=w348:string)
        n213 = call-dynamic "Enable Control.vi"("Select Channel"=w352, "Enable Control"=w351, "Temp Control in"=w361) -> ("Temp Control out"=w360:refnum<class "Temp Control.lvclass">)  [unwired: 7 in, 1 out]
        n214 = Format Into String(format string="Temperature control %s on channel %d", w348, w352) -> (resulting string=w353:string)  [unwired: 2 in, 1 out]
        n215 = Bundle By Name(cluster=w358, "Temp Control ref"=w360) -> (w359:T6)
        n216 = call "Temp Control Message Log.vi"("String in"=w353) -> ()  [unwired: 9 in, 2 out]
      }
      event "Setpoint 1", "Setpoint 2": Value Change {
        n217 = event-data() -> ("CtlRef"=w371:refnum<vi>)  [unwired: 1 in, 5 out]
        n218 = property class="DigNum (strict)"(reference=w371) -> ("Label.Text"=w370:string)  [unwired: 1 in, 2 out]
        n219 = case shown="\"False\", Default" w370 {
          tunnel: ["Setpoint 1" "Setpoint 2"] -> w366
          tunnel: [1 2] -> w367
          frame "False", Default {
          }
          frame "Setpoint 2" {
          }
        }
        n220 = Unbundle By Name(w374) -> ("Temp Control ref"=w373:refnum<class "Temp Control.lvclass">)
        n221 = call-dynamic "Set Setpoint.vi"("Select Channel"=w367, "Setpoint"=w366, "Temp Control in"=w373) -> ("Temp Control out"=w372:refnum<class "Temp Control.lvclass">)  [unwired: 7 in, 1 out]
        n222 = Bundle By Name(cluster=w374, "Temp Control ref"=w372) -> (w375:T6)
        n223 = Format Into String(format string="Temperature control channel %d set to %f", w367, w366) -> (resulting string=w368:string)  [unwired: 2 in, 1 out]
        n224 = call "Temp Control Message Log.vi"("String in"=w368) -> ()  [unwired: 9 in, 2 out]
      }
      event "Standalone": Value Change {
        n225 = event-data() -> ("NewVal"=w380:bool)  [unwired: 1 in, 5 out]
        n226 = property on="Close" class="Bool"("Visible"=w380) -> ()  [unwired: 2 in, 2 out]
      }
      event "Status": Value Change {
        n227 = event-data() -> ("NewVal"=w385:i32[])  [unwired: 1 in]
        n228 = Unbundle By Name(w382) -> ("Temp Control ref"=w387:refnum<class "Temp Control.lvclass">, "Buffer"=w389:refnum<class "Data Buffer.lvclass">)
        n229 = call-dynamic "read buffer.vi"("Data Buffer in"=w389) -> ("XY Graph"=w388:T3)  [unwired: 8 in, 2 out]
        n230 = for {
          tunnel: w385 -> [w394] mode=indexing
          tunnel: w388 -> [w395]
          tunnel: [w393] -> w392 mode=indexing
          n231 = Index Array(array=w395, index=w394) -> (element=w393:T14)
        }
        n232 = call-dynamic "Write Ch Select.vi"("Ch Select"=w385, "Temp Control in"=w387) -> ("Temp Control out"=w386:refnum<class "Temp Control.lvclass">)  [unwired: 8 in, 1 out]
        n233 = call-dynamic "Read Channel Names.vi"("Temp Control in"=w386) -> ("Channel Names"=w390:string[], "Temp Control out"=w384:refnum<class "Temp Control.lvclass">)  [unwired: 8 in, 1 out]
        n234 = property on="XY Graph" class="XYGraph (strict)"("Value"=w392) -> (error out=w391:errorcluster)  [unwired: 2 in, 1 out]
        n235 = Bundle By Name(cluster=w382, "Temp Control ref"=w384) -> (w383:T6)
        n236 = for {
          N -> [w396]
          tunnel: w385 -> [w400] mode=indexing
          tunnel: w390 -> [w401]
          tunnel: w391 -> [w397]
          i -> [w399]
          n237 = Index Array(array=w401, index=w400) -> (element=w398:string)
          n238 = property on="XY Graph" class="XYGraph (strict)"(error in=w397, "Active Plot"=w399, "Plot.Plot Name"=w398, "LegNumRows"=w396) -> ()  [unwired: 1 in, 2 out]
        }
      }
      event "Tempcontrol Type": Value Change {
        n239 = event-data() -> ("CtlRef"=w410:refnum<vi>)  [unwired: 1 in, 5 out]
        n240 = property class="Ring (strict)"(reference=w410) -> ("Strings []"=w409:string[])  [unwired: 1 in, 2 out]
        n241 = Unbundle By Name(w406) -> ("state"=w405:refnum<user-event>)
        n242 = Generate User Event(user event=w405, event data cluster="Reinit" ("event data")) -> ()  [unwired: 2 in, 2 out]
        n243 = Index Array(array=w409, index="Tempcontrol Type") -> (element=w402:string)
        n244 = call "CC Set Device By Name.vi"("Device Name"=w402, "Device Type"="Temp Control") -> ()  [unwired: 8 in, 2 out]
        n245 = Bundle By Name(cluster=w406, "Device"=w402) -> (w407:T6)
      }
      event "Addr": Value Change {
        n246 = event-data() -> ()  [unwired: 1 in, 6 out]
        n247 = Unbundle By Name(w411) -> ("state"=w417:refnum<user-event>, "Temp Control ref"=w415:refnum<class "Temp Control.lvclass">)
        n248 = Generate User Event(user event=w417, event data cluster="Reinit" ("event data")) -> ()  [unwired: 2 in, 2 out]
        n249 = call-dynamic "Write Addr.vi"("Addr"="Addr", "Temp Control in"=w415) -> ("Temp Control out"=w413:refnum<class "Temp Control.lvclass">)  [unwired: 8 in, 1 out]
        n250 = Bundle By Name(cluster=w411, "Temp Control ref"=w413) -> (w412:T6)
      }
      event "Reinit": Value Change {
        n251 = event-data() -> ()  [unwired: 1 in, 6 out]
        n252 = Unbundle By Name(w418) -> ("state"=w420:refnum<user-event>)
        n253 = Generate User Event(user event=w420, event data cluster="Reinit" ("event data")) -> ()  [unwired: 2 in, 2 out]
      }
      event Value Change {
        n254 = event-data() -> ()  [unwired: 1 in, 6 out]
        n255 = case shown="\"User\", Default" "Mode" {
          tunnel: [bool[] [TRUE, FALSE, FALSE] bool[] [TRUE, TRUE, TRUE]] -> w421
          frame "User", Default {
          }
          frame "Engineering" {
          }
        }
        n256 = property on="Tab Control" class="TabCtl (strict)"() -> ("Pages"=w422:refnum<vi>[])  [unwired: 2 in, 2 out]
        n257 = for {
          tunnel: w422 -> [w426] mode=indexing
          tunnel: w421 -> [w425] mode=indexing
          n258 = property class="Page"(reference=w426, "PageVis"=w425) -> ()  [unwired: 1 in, 2 out]
        }
      }
      event "Close": Value Change {
        n259 = event-data() -> ()  [unwired: 1 in, 2 out]
        n260 = Unbundle By Name(w431) -> ("state"=w430:refnum<user-event>)
        n261 = Generate User Event(user event=w430, event data cluster="Shutdown" ("event data")) -> ()  [unwired: 2 in, 2 out]
      }
    }
  }
